vi "Test_RouteGuide_Unary.vi"() -> (0 "Array of Error Description":T1)   [LabVIEW 2025]
uses:
  gRPC_ATS/TestUtility/utility.llb/array of error description.ctl
  gRPC_ATS/TestUtility/utility.llb/error description.ctl
  gRPC_ATS/TestUtility/utility.llb/error type.ctl
  examples/route_guide/route_guide_client/RPC Messages/routeguide_Feature.ctl
  examples/route_guide/route_guide_client/RPC Messages/routeguide_Point.ctl
  examples/route_guide/route_guide_client/route_guide_client.lvlib
panel:
  out "Pass":bool
  in  "Client VI Path":path=path "../../examples/route_guide/route_guide_client/Unary RouteGuide Test.vi"
  in  "Server VI path":path=path "../../examples/route_guide/route_guide_server/Run Service.vi"
  in  "error in":errorcluster
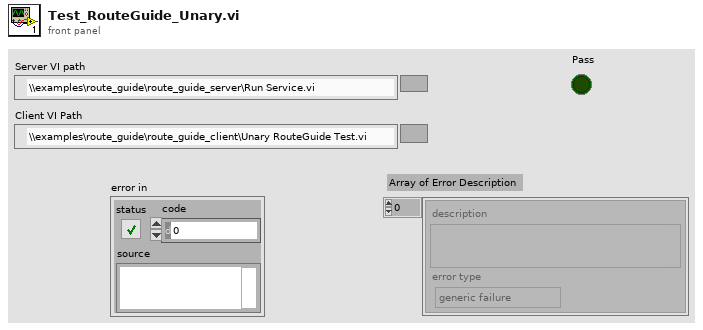
[diagram p1: front panel]
types:
  T1 = typedef "array of error description.ctl" = T2[]
  T2 = typedef "error description.ctl" = cluster{"description":string, "error type":T3}
  T3 = typedef "error type.ctl" = enum32{"generic failure", "boundary case", "precision", "expected error"}
  T4 = typedef "route_guide_client.lvlib/routeguide_Feature.ctl" = cluster{"name":string, "location":T5}
  T5 = typedef "route_guide_client.lvlib/routeguide_Point.ctl" = cluster{"latitude":i32, "longitude":i32}
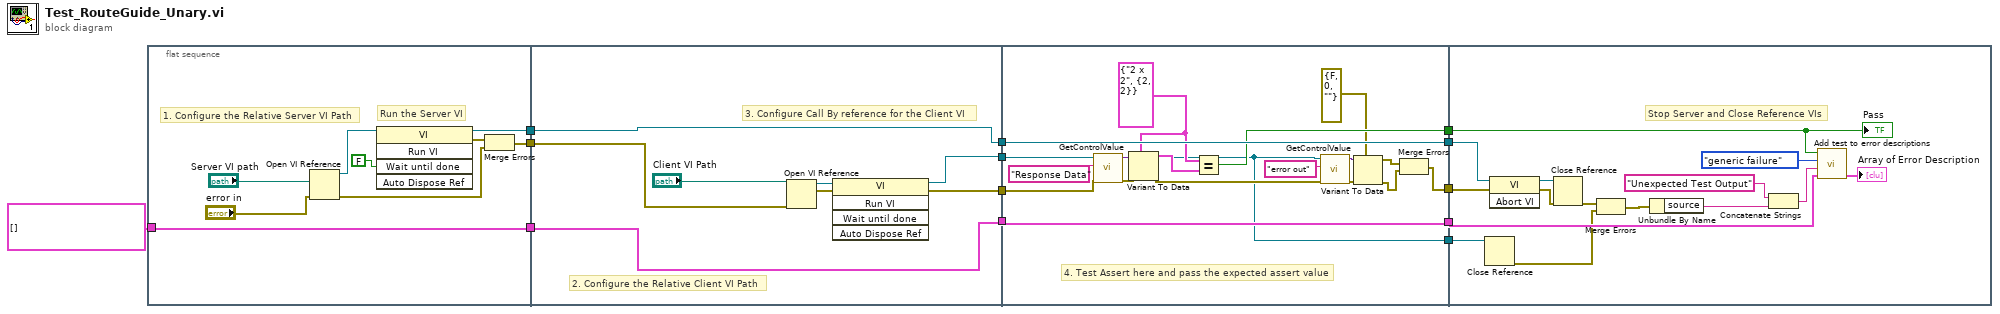
[diagram p0: block diagram]
diagram:
  n1 = flat-sequence {
    tunnel: T1 [] ("error descriptions in") -> [w18]
    tunnel: [w18] -> w13
    tunnel: [w17] -> w12
    tunnel: [w14] -> w11
    tunnel: w13 -> [w29]
    tunnel: [w29] -> w10
    tunnel: [w28] -> w9
    tunnel: w12 -> [w28]
    tunnel: w11 -> [w27]
    tunnel: [w24] -> w4
    tunnel: [w23] -> w3
    tunnel: w10 -> [w48]
    tunnel: [w48] -> w8
    tunnel: [w47] -> w7
    tunnel: w9 -> [w47]
    tunnel: [w46] -> w5
    tunnel: w4 -> [w32]
    tunnel: w3 -> [w37]
    tunnel: [w33] -> w2
    tunnel: [w32] -> w1
    tunnel: w8 -> [w58]
    tunnel: w7 -> [w55]
    tunnel: w5 -> [w53]
    tunnel: w2 -> [w54]
    tunnel: w1 -> [w49]
    frame #0 {
      # "1. Configure the Relative Server VI Path"
      # "Run the Server VI"
      n2 = Open VI Reference(vi path="Server VI path", error in (no error)="error in") -> (vi reference=w20:refnum<vi>, error out=w16:errorcluster)  [unwired: 4 in]
      n3 = invoke class="VI" method="Run VI"(reference=w20, "Wait until done"=FALSE ("Wait Until Done")) -> (reference out=w17:refnum<vi>, error out=w15:errorcluster)  [unwired: 3 in, 3 out]
      n4 = Merge Errors(w15, w16) -> (w14:errorcluster)
    }
    frame #1 {
      # "2. Configure the Relative Client VI Path"
      # "3. Configure Call By reference for the Client VI"
      n5 = Open VI Reference(vi path="Client VI Path", error in (no error)=w27) -> (vi reference=w26:refnum<vi>, error out=w25:errorcluster)  [unwired: 4 in]
      n6 = invoke class="VI" method="Run VI"(reference=w26, error in=w25) -> (reference out=w24:refnum<vi>, error out=w23:errorcluster)  [unwired: 3 in, 3 out]
    }
    frame #2 {
      w42 = T4 {"name"="2 x 2", "location"={"latitude"=2, "longitude"=2}} ("Response Data")
      # "4. Test Assert here and pass the expected assert value"
      n7 = call "GetControlValue.vi"("error in (no error)"=w37, "Control Label"="Response Data", "VI Reference"=w32) -> ("error out"=w44:errorcluster, "Value"=w43:variant)  [unwired: 7 in]
      n8 = Variant To Data(error in=w44, type=w42, Variant=w43) -> (data=w41:T4, error out=w36:errorcluster)
      n9 = Equal?(x=w42, y=w41) -> (x = y?=w46:bool)
      n10 = call "GetControlValue.vi"("error in (no error)"=w36, "Control Label"="error out", "VI Reference"=w32) -> ("error out"=w39:errorcluster, "Value"=w31:variant)  [unwired: 7 in]
      n11 = Variant To Data(error in=w39, type=errorcluster {"status"=FALSE, "code"=0, "source"=""} ("error constant"), Variant=w31) -> (data=w35:errorcluster, error out=w34:errorcluster)
      n12 = Merge Errors(w35, w34) -> (w33:errorcluster)
    }
    frame #3 {
      # "Stop Server and Close Reference VIs"
      n13 = Close Reference(reference=w49) -> (error out=w51:errorcluster)  [unwired: 1 in]
      n14 = invoke class="VI" method="Abort VI"(reference=w55, error in=w54) -> (reference out=w56:refnum<vi>, error out=w57:errorcluster)  [unwired: 1 in, 1 out]
      n15 = Close Reference(reference=w56, error in (no error)=w57) -> (error out=w52:errorcluster)
      n16 = Merge Errors(w52, w51) -> (w50:errorcluster)
      n17 = Unbundle By Name(w50) -> ("source"=w60:string)
      n18 = Concatenate Strings("Unexpected Test Output" ("string"), w60) -> (w61:string)
      n19 = call "Add test to error descriptions.vi"("error descriptions in"=w58, "error string"=w61, "error type"=error_type."generic failure", "pass"=w53) -> ("error description out"=→"Array of Error Description":T1)  [unwired: 3 in]
      "Pass" <- w53
    }
  }
